vi "MSC Type to IMAQ Type.vi"(0 "MSC Picture Type":T2 items=["Grayscale U8"=0, "Grayscale U16"=2, "Grayscale Single"=5, "Grayscale Double"=6, "RGB U8"=16], 11 "error in (no error)":errorcluster) -> (4 "IMAQ Type":T1 items=["Grayscale (U8)", "Grayscale (I16)", "Grayscale (SGL)", "Complex (CSG)", "RGB (U32)", "HSL (U32)", "RGB (U64)", "Grayscale (U16)"], 15 "error out":errorcluster)   [LabVIEW 2016]
doc: "Conversion from MSC Picture type to IMAQ type"
uses:
  MSC Image_class/controls/Image Type.ctl
  MSC Image_class/MSC Image.lvclass
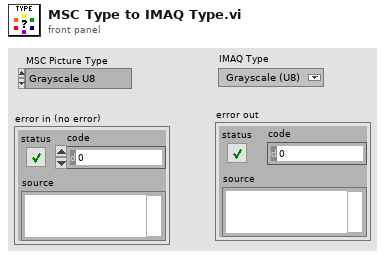
[diagram p1: front panel]
types:
  T1 = typedef "Image Type" = u32
  T2 = typedef "MSC Image.lvclass/Image Type.ctl" = i32
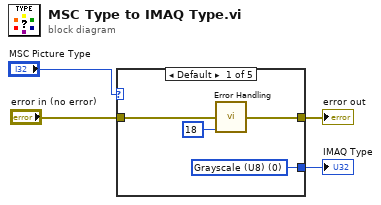
[diagram p0: block diagram]
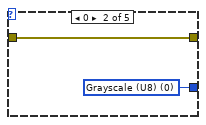
[diagram p2: hidden frame]
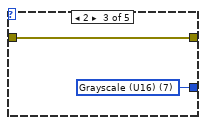
[diagram p3: hidden frame]
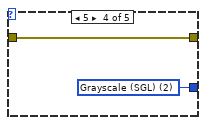
[diagram p4: hidden frame]
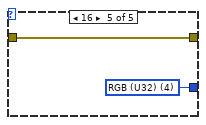
[diagram p5: hidden frame]
diagram:
  n1 = case shown="Default" "MSC Picture Type" {
    tunnel: "error in (no error)" -> [w7 w10 w12 w14 w16]
    tunnel: [w5 w10 w12 w14 w16] -> w3
    tunnel: [w8 w9 w11 w13 w15] -> w2
    frame Default {
      w8 = T1 0 items=["Grayscale (U8)", "Grayscale (I16)", "Grayscale (SGL)", "Complex (CSG)", "RGB (U32)", "HSL (U32)", "RGB (U64)", "Grayscale (U16)"] ("IMAQ Type")
      n2 = call "Error Handling.vi"("error in (no error)"=w7, "return type"=18 ("code")) -> ("error out"=w5:errorcluster)  [unwired: 12 in, 1 out]
    }
    frame 0 {
      w9 = T1 0 items=["Grayscale (U8)", "Grayscale (I16)", "Grayscale (SGL)", "Complex (CSG)", "RGB (U32)", "HSL (U32)", "RGB (U64)", "Grayscale (U16)"] ("IMAQ Type")
    }
    frame 2 {
      w11 = T1 7 items=["Grayscale (U8)", "Grayscale (I16)", "Grayscale (SGL)", "Complex (CSG)", "RGB (U32)", "HSL (U32)", "RGB (U64)", "Grayscale (U16)"] ("IMAQ Type")
    }
    frame 5 {
      w13 = T1 2 items=["Grayscale (U8)", "Grayscale (I16)", "Grayscale (SGL)", "Complex (CSG)", "RGB (U32)", "HSL (U32)", "RGB (U64)", "Grayscale (U16)"] ("IMAQ Type")
    }
    frame 16 {
      w15 = T1 4 items=["Grayscale (U8)", "Grayscale (I16)", "Grayscale (SGL)", "Complex (CSG)", "RGB (U32)", "HSL (U32)", "RGB (U64)", "Grayscale (U16)"] ("IMAQ Type")
    }
  }
  "IMAQ Type" <- w2
  "error out" <- w3
